vi "TangoConnect.vi"(9 "show Protocol":bool, 11 "Tango Com":refnum<visa-resource-name>) -> (0 "error out":errorcluster, 2 "success":bool, 3 "plLSID out":i32, 10 "Baud":dbl)   [LabVIEW 2018, in "TangoOWN.lvlib"]
uses:
  TangoOWN.lvlib
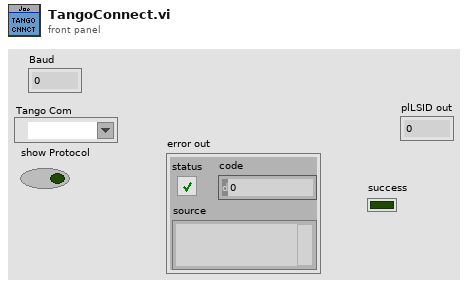
[diagram p1: front panel]
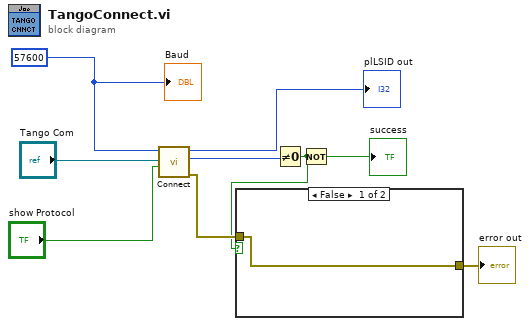
[diagram p0: block diagram]
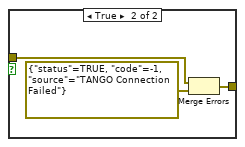
[diagram p2: hidden frame]
diagram:
  w9 = 57600 ("lABaudRate")
  n1 = call "Connect.vi"("ShProt?"="show Protocol", "pcAComName"="Tango Com", "lABaudRate"=w9) -> ("error out"=w3:errorcluster, "function return"=w6:i32, "plLSID out"=→"plLSID out":i32)  [unwired: 5 in]
  n2 = Not Equal To 0?(x=w6) -> (x != 0?=w1:bool)
  n3 = case shown="False" w1 {
    tunnel: w3 -> [w10 w12]
    tunnel: [w10 w11] -> w2
    frame False {
    }
    frame True {
      n4 = Merge Errors(w12, errorcluster {"status"=TRUE, "code"=-1, "source"="TANGO Connection Failed"} ("error constant")) -> (w11:errorcluster)
    }
  }
  "error out" <- w2
  n5 = Not(x=w1) -> (.not. x?=→"success":bool)
  "Baud" <- w9
